vi "PLC_to_Auto.vi"() -> ()   [LabVIEW 2017]
panel:
  out "PLC Communication STATION 1":bool
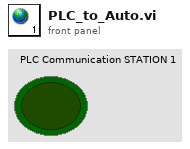
[diagram p1: front panel]
diagram:
